vi "thermometer_controller.vi"(8 "error in (no error)":errorcluster, 11 "module name":string) -> (0 "error out":errorcluster)   [LabVIEW 2019]
uses:
  thermometer1/thermometer1 support vi/thermometer1_units.ctl
  common/common data types/common_event_data.ctl
panel:
  out "target thermometer temp":dbl(slide) scale=0.0..100.0
  in  "Sample rate (1-100 Hz)":dbl(knob)=20.0 min=1.0 max=100.0 step=1.0 scale=1.0..100.0
  in  "units":T1
  in  "target thermometer":string="thermometer1"
  out "global stop?":bool
  in  "stop this module":bool
  out "targetted":bool
  out "target":string
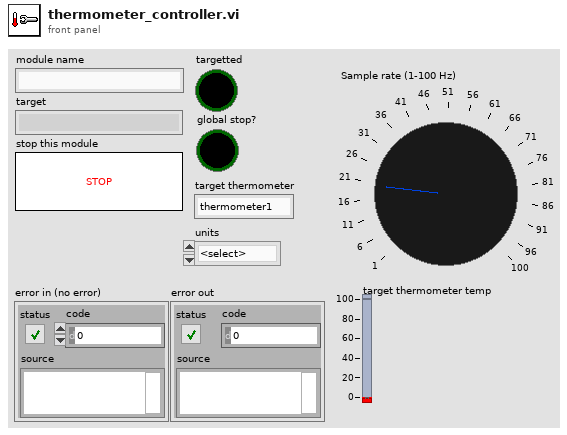
[diagram p1: front panel]
types:
  T1 = typedef "thermometer1_units.ctl" = enum16{"<select>", "C", "F", "K"}
  T2 = typedef "common_event_data.ctl" = cluster{"sender":string, "target":string, "msg":string, "data":variant}
  T3 = cluster{"module name":string, "example data":bool}
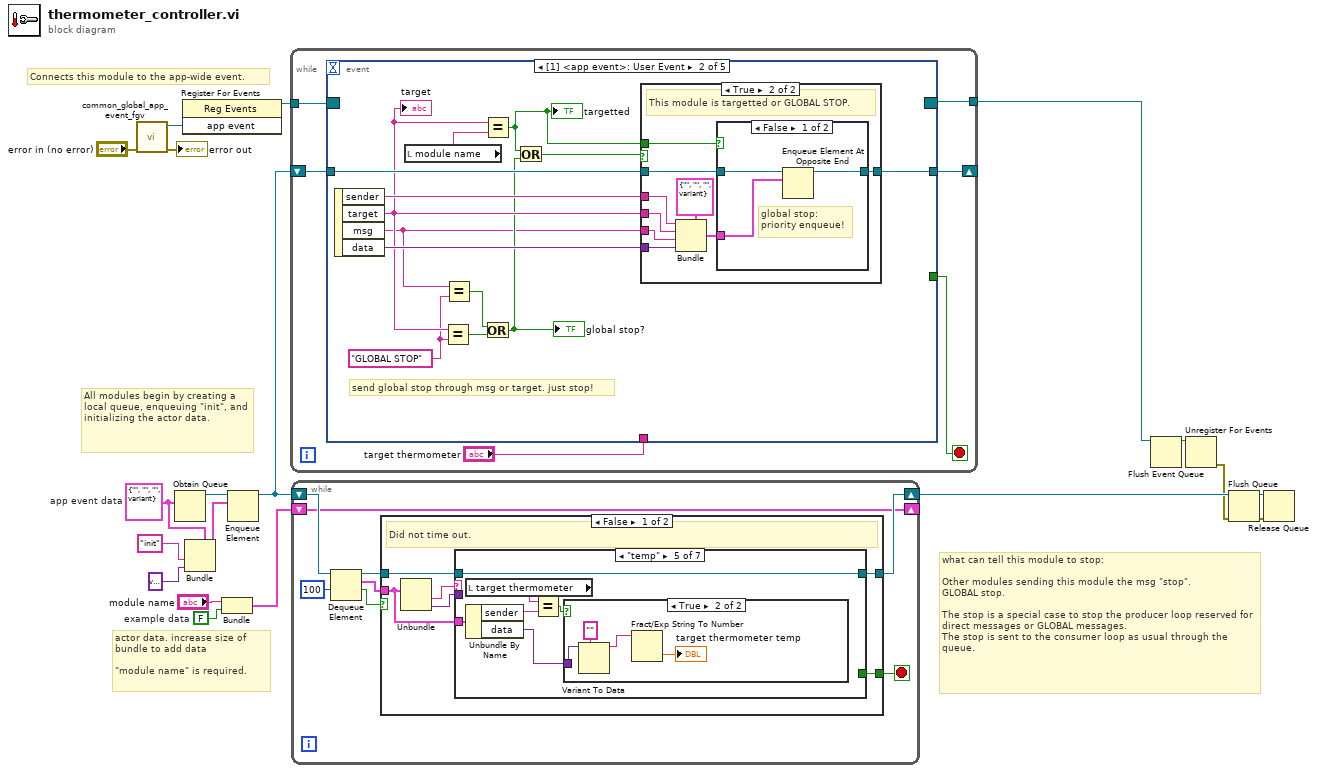
[diagram p0: block diagram]
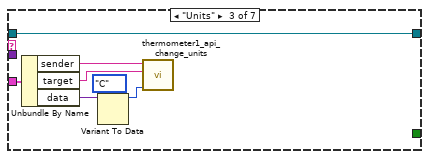
[diagram p4: hidden frame]
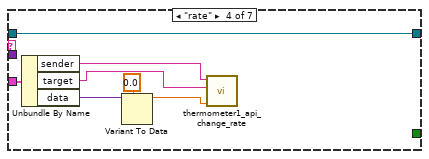
[diagram p5: hidden frame]
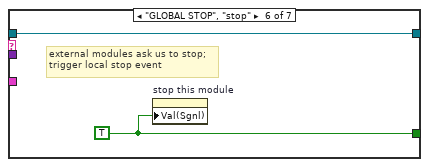
[diagram p7: hidden frame]
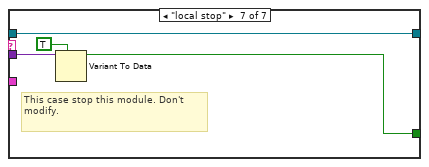
[diagram p8: hidden frame]
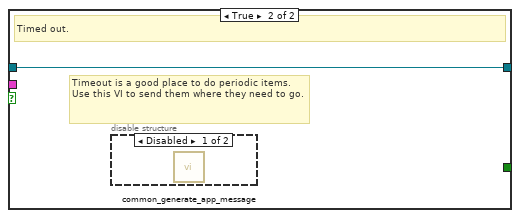
[diagram p9: hidden frame]
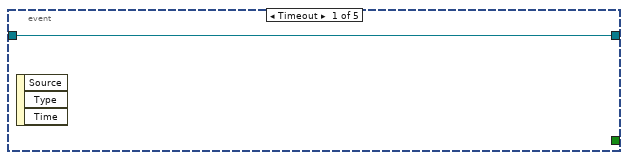
[diagram p11: hidden frame]
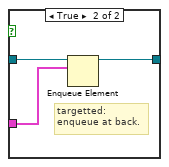
[diagram p13: hidden frame]
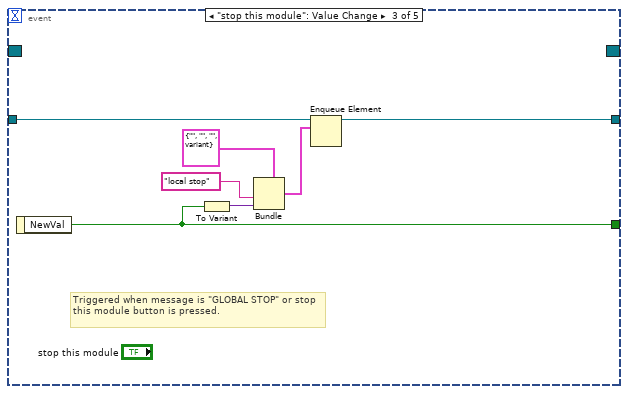
[diagram p14: hidden frame]
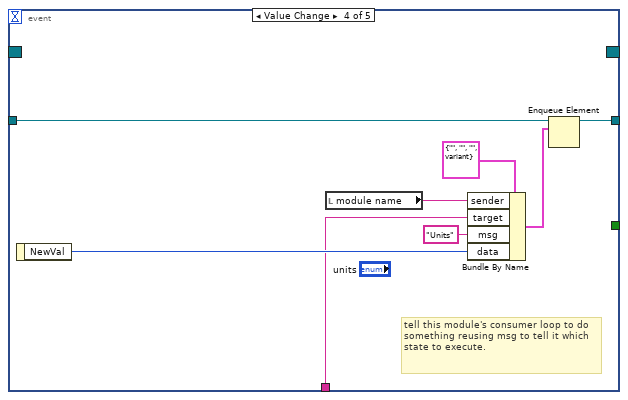
[diagram p15: hidden frame]
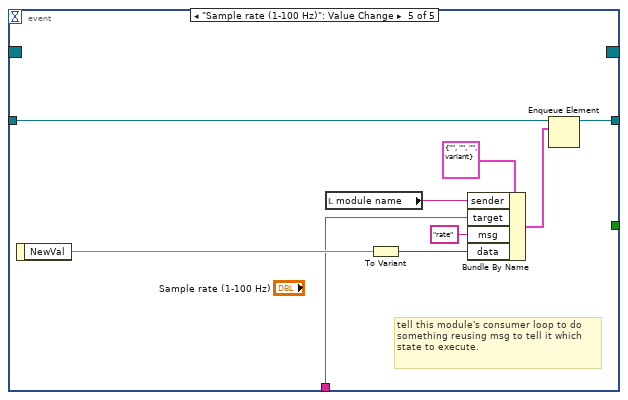
[diagram p16: hidden frame]
diagram:
  w5 = FALSE  # example data
  w8 = T2 {"sender"="", "target"="", "msg"="", "data"=variant}  # app event data
  # "All modules begin by creating a local queue, enqueuing \"init\", and initializing the actor data."
  # "actor data. increase size of bundle to add data\n\n\"module name\" is required."
  # "what can tell this module to stop:\n\nOther modules sending this module the msg \"stop\".\nGLOBAL stop.\n\nThe stop is a special case to stop the producer loop reserved for direct messages or GLOBAL messages.\nThe stop is sent to the consumer loop as usual through the queue."
  # "Connects this module to the app-wide event."
  n1 = call "common_global_app_event_fgv.vi"("error in (no error)"="error in (no error)") -> ("error out"=→"error out":errorcluster, "app event"=w13:refnum<user-event>)  [unwired: 9 in]
  n2 = Obtain Queue(element data type=w8) -> (queue out=w19:refnum<queue>)  [unwired: 4 in, 2 out]
  n3 = register-events(w13) -> (reference out=w14:refnum<event-registration>)  [unwired: 2 in, 1 out]
  n4 = Bundle(cluster=w8, "msg"="init", "data"=variant) -> (w18:T2)  [unwired: 2 in]
  n5 = Bundle("module name"="module name", "example data"=w5) -> (w4:T3)  [unwired: 1 in]
  n6 = Enqueue Element(queue=w19, element=w18) -> (queue out=w17:refnum<queue>)  [unwired: 2 in, 2 out]
  n7 = while {
    tunnel: w14 -> [w25]
    shift-right: [w23] -> _
    shift-left: w17 -> [w24]
    tunnel: [w22] -> w3
    stop <- w21 stop-if-true
    n8 = event shown="[1] <app event>: User Event" {
      selector: w25 -> [_ _ _ _ _]
      dyn-events: [_ _ _ _ _] -> w22
      timeout: _ -> [_ _ _ _ _]
      tunnel: w24 -> [w26 w38 w60 w69 w78]
      tunnel: [w26 w37 w61 w70 w79] -> w23
      tunnel: [_ _ w56 _ _] -> w21
      tunnel: "target thermometer" -> [_ _ _ w63 w71]
      event Timeout {
        n9 = event-data() -> ()  [unwired: 1 in, 3 out]
      }
      event User Event {
        w30 = "GLOBAL STOP"
        # "send global stop through msg or target. just stop!"
        n10 = event-data() -> ("sender"=w36:string, "target"=w35:string, "msg"=w29:string, "data"=w39:variant)  [unwired: 1 in]
        "target" <- w35
        n11 = local read "module name"() -> (w27:string)
        n12 = Equal?(x=w35, y=w30) -> (x = y?=w32:bool)
        n13 = Equal?(x=w29, y=w30) -> (x = y?=w28:bool)
        n14 = Equal?(x=w35, y=w27) -> (x = y?=w33:bool)
        "targetted" <- w33
        n15 = Or(x=w28, y=w32) -> (x .or. y?=w31:bool)
        "global stop?" <- w31
        n16 = Or(x=w33, y=w31) -> (x .or. y?=w34:bool)
        n17 = case shown="True" w34 {
          tunnel: w29 -> [_ w45]
          tunnel: w39 -> [_ w46]
          tunnel: w38 -> [w40 w49]
          tunnel: [w40 w48] -> w37
          tunnel: w35 -> [_ w44]
          tunnel: w36 -> [_ w43]
          tunnel: w33 -> [_ w41]
          frame False {
          }
          frame True {
            # "This module is targetted or GLOBAL STOP."
            n18 = Bundle(cluster=T2 {"sender"="", "target"="", "msg"="", "data"=variant}, "sender"=w43, "target"=w44, "msg"=w45, "data"=w46) -> (w42:T2)
            n19 = case shown="False" w41 {
              tunnel: w49 -> [w52 w55]
              tunnel: [w51 w54] -> w48
              tunnel: w42 -> [w50 w53]
              frame False {
                # "global stop:\npriority enqueue!"
                n20 = Enqueue Element At Opposite End(queue=w52, element=w50) -> (queue out=w51:refnum<queue>)  [unwired: 2 in, 2 out]
              }
              frame True {
                # "targetted:\nenqueue at back."
                n21 = Enqueue Element(queue=w55, element=w53) -> (queue out=w54:refnum<queue>)  [unwired: 2 in, 2 out]
              }
            }
          }
        }
      }
      event "stop this module": Value Change {
        # "Triggered when message is \"GLOBAL STOP\" or stop this module button is pressed."
        n22 = event-data() -> ("NewVal"=w56:bool)  [unwired: 1 in]
        n23 = To Variant(anything=w56) -> (Variant=w57:variant)
        n24 = Bundle(cluster=T2 {"sender"="", "target"="", "msg"="", "data"=variant}, "msg"="local stop", "data"=w57) -> (w62:T2)  [unwired: 2 in]
        n25 = Enqueue Element(queue=w60, element=w62) -> (queue out=w61:refnum<queue>)  [unwired: 2 in, 2 out]
      }
      event Value Change {
        # "tell this module's consumer loop to do something reusing msg to tell it which state to execute."
        n26 = event-data() -> ("NewVal"=w67:T1)  [unwired: 1 in]
        n27 = local read "module name"() -> (w66:string)
        n28 = Bundle By Name(cluster=T2 {"sender"="", "target"="", "msg"="", "data"=variant} ("element"), "sender"=w66, "target"=w63, "msg"="Units", "data"=w67) -> (w64:T2)
        n29 = Enqueue Element(queue=w69, element=w64) -> (queue out=w70:refnum<queue>)  [unwired: 2 in, 2 out]
      }
      event "Sample rate (1-100 Hz)": Value Change {
        # "tell this module's consumer loop to do something reusing msg to tell it which state to execute."
        n30 = event-data() -> ("NewVal"=w73:dbl)  [unwired: 1 in]
        n31 = local read "module name"() -> (w74:string)
        n32 = To Variant(anything=w73) -> (Variant=w72:variant)
        n33 = Bundle By Name(cluster=T2 {"sender"="", "target"="", "msg"="", "data"=variant} ("element"), "sender"=w74, "target"=w71, "msg"="rate", "data"=w72) -> (w75:T2)
        n34 = Enqueue Element(queue=w78, element=w75) -> (queue out=w79:refnum<queue>)  [unwired: 2 in, 2 out]
      }
    }
  }
  n35 = while {
    shift-right: [w84] -> w15
    shift-left: w17 -> [w87]
    shift-right: [w80] -> _
    shift-left: w4 -> [w80]
    stop <- w83 stop-if-true
    n36 = Dequeue Element(queue=w87, timeout in ms (-1)=100) -> (queue out=w85:refnum<queue>, element=w86:T2, timed out?=w82:bool)  [unwired: 1 in, 1 out]
    n37 = case shown="False" w82 {
      tunnel: w86 -> [w88 _]
      tunnel: w85 -> [w93 w126]
      tunnel: [w92 w126] -> w84
      tunnel: [w91 _] -> w83
      frame False {
        # "Did not time out."
        n38 = Unbundle(w88) -> ("msg"=w89:string, "data"=w90:variant)  [unwired: 2 out]
        n39 = case shown="\"temp\"" w89 {
          tunnel: w93 -> [w94 w95 w102 w109 w113 w121 w125]
          tunnel: [w94 w95 w102 w109 w113 w121 w125] -> w92
          tunnel: w90 -> [_ _ _ _ _ _ w123]
          tunnel: [_ _ _ _ _ w120 w122] -> w91
          tunnel: w88 -> [_ _ w101 w108 w115 _ _]
          frame Default {
            # "unsupported message."
          }
          frame "init" {
          }
          frame "Units" {
            n40 = Unbundle By Name(w101) -> ("sender"=w100:string, "target"=w99:string, "data"=w97:variant)
            n41 = Variant To Data(type=thermometer1_units."C" ("units"), Variant=w97) -> (data=w96:T1)  [unwired: 1 in, 1 out]
            n42 = call "thermometer1_api_change_units.vi"("units"=w96, "target (\"thermometer1\")"=w99, "sender"=w100) -> ()  [unwired: 9 in]
          }
          frame "rate" {
            n43 = Unbundle By Name(w108) -> ("sender"=w106:string, "target"=w105:string, "data"=w107:variant)
            n44 = Variant To Data(type=0.0 ("Sample rate (1-100 Hz)"), Variant=w107) -> (data=w103:dbl)  [unwired: 1 in, 1 out]
            n45 = call "thermometer1_api_change_rate.vi"("Sample rate (1-100 Hz)"=w103, "target (\"thermometer1\")"=w105, "sender"=w106) -> ()  [unwired: 9 in]
          }
          frame "temp" {
            n46 = local read "target thermometer"() -> (w110:string)
            n47 = Unbundle By Name(w115) -> ("sender"=w111:string, "data"=w114:variant)
            n48 = Equal?(x=w110, y=w111) -> (x = y?=w112:bool)
            n49 = case shown="True" w112 {
              tunnel: w114 -> [_ w119]
              frame False {
              }
              frame True {
                n50 = Variant To Data(type="", Variant=w119) -> (data=w116:string)  [unwired: 1 in, 1 out]
                n51 = Fract/Exp String To Number(string=w116) -> (number=→"target thermometer temp":dbl)  [unwired: 3 in, 1 out]
              }
            }
          }
          frame "GLOBAL STOP", "stop" {
            w120 = TRUE
            # "external modules ask us to stop;\ntrigger local stop event"
            n52 = property on="stop this module" class="Bool (strict)"("Val(Sgnl)"=w120) -> ()  [unwired: 2 in, 2 out]
          }
          frame "local stop" {
            # "This case stop this module. Don't modify."
            n53 = Variant To Data(type=TRUE, Variant=w123) -> (data=w122:bool)  [unwired: 1 in, 1 out]
          }
        }
      }
      frame True {
        # "Timeout is a good place to do periodic items. Use this VI to send them where they need to go."
        # "Timed out."
        n54 = disable-structure shown="Disabled" {
          frame Disabled {
            n55 = call "common_generate_app_message.vi"() -> ()  [unwired: 11 in, 1 out]
          }
          frame Enabled {
          }
        }
      }
    }
  }
  n56 = Flush Event Queue(0:w3) -> (8:w2:refnum<event-registration>)  [unwired: 5 in, 2 out]
  n57 = Unregister For Events(event registration refnum=w2) -> (error out=w10:errorcluster)  [unwired: 1 in]
  n58 = Flush Queue(queue=w15, error in (no error)=w10) -> (queue out=w16:refnum<queue>, error out=w9:errorcluster)  [unwired: 1 out]
  n59 = Release Queue(queue=w16, error in (no error)=w9) -> ()  [unwired: 1 in, 3 out]
